vi "Euler_matrix (SubVI).vi"(11 "Special Matrix":T1) -> (3 "eual_matrix":T1)   [LabVIEW 2018]
uses:
  <vilib>/Analysis/Matrix/Datatypes/RealMatrix.ctl
  <vilib>/Analysis/NI_AALPro.lvlib
  <vilib>/Analysis/Matrix/NI_Matrix.lvlib
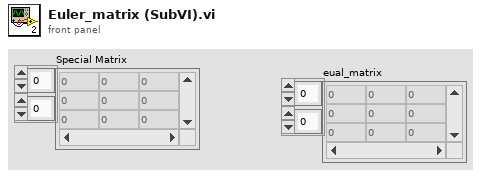
[diagram p1: front panel]
types:
  T1 = typedef "NI_Matrix.lvlib/RealMatrix.ctl" = dbl[][]
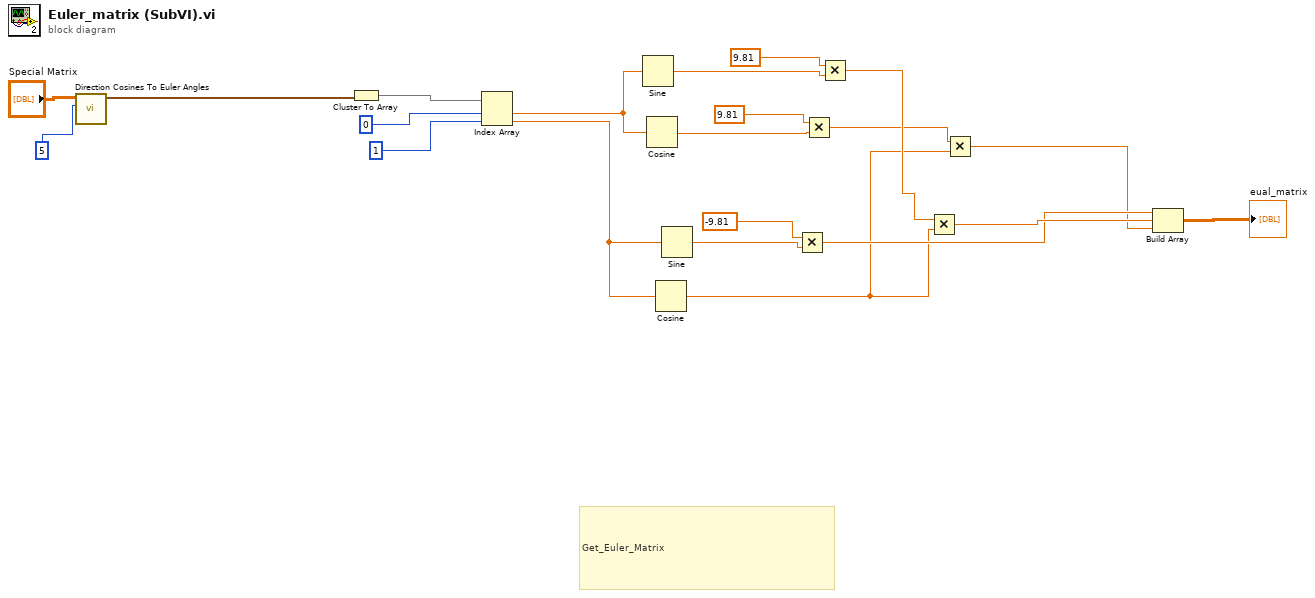
[diagram p0: block diagram]
diagram:
  # "Get_Euler_Matrix"
  n1 = call <vilib>:"Direction Cosines To Euler Angles.vi"("rotation order"=5, "Direction Cosines"="Special Matrix") -> ("Euler Angles"=w18:cluster{"phi":dbl, "theta":dbl, "psi":dbl})  [unwired: 8 in, 1 out]
  n2 = Cluster To Array(cluster=w18) -> (array=w19:dbl[])
  n3 = Index Array(array=w19, index #1=0, index #2=1) -> (element #1=w14:dbl, element #2=w15:dbl)
  n4 = Sine(x=w14) -> (sin(x)=w8:dbl)
  n5 = Cosine(x=w14) -> (cos(x)=w12:dbl)
  n6 = Cosine(x=w15) -> (cos(x)=w3:dbl)
  n7 = Sine(x=w15) -> (sin(x)=w10:dbl)
  n8 = Multiply(x=-9.81, y=w10) -> (x*y=w5:dbl)
  n9 = Multiply(x=9.81, y=w12) -> (x*y=w4:dbl)
  n10 = Multiply(x=9.81, y=w8) -> (x*y=w7:dbl)
  n11 = Multiply(x=w7, y=w3) -> (x*y=w6:dbl)
  n12 = Multiply(x=w4, y=w3) -> (x*y=w2:dbl)
  n13 = Build Array(w5, w6, w2) -> (→"eual_matrix":T1)
